vi "img test14(coutsegment attempt2).vi"() -> ()   [LabVIEW 2013]
uses:
  <vilib>/vision/NI_Vision_Development_Module.lvlib
panel:
  out "Top player court segment display 2":bool[][](array[boolean])
  out "count top":i32[](graph)
  out "count bottom":i32[](graph)
  out "trans top":i32[](graph)
  out "trans bottom":i32[](graph)
  out "trans array bottom":i32[](array[numeric])
  out "trans array top":i32[](array[numeric])
  out "count array bottom":i32[](array[numeric])
  out "Count array top":i32[](array[numeric])
  in  "ON":bool
  out "Top player court segment display":bool[][](array[boolean])
  out "bottom player":cluster{"Numeric":dbl, "Numeric":dbl}[](array[cluster])
  out "top player":cluster{"Numeric":dbl, "Numeric":dbl}[](array[cluster])
  in  "playing":bool
  out "Top VIew":cluster{"Numeric":dbl, "Numeric":dbl}[](graph)
  out "Image 4":T1(plugin-control)
  in  "frame jump":i32=3
  in  "speed":u32(slide)
  in  "start":i32(slide) step=219843704 scale=0.0..5867.0
  out "Image 3":T1(plugin-control)
  in  "AVI Path":path=path "E:/PhD work/Videos/ChenJin vs HuYun.avi"
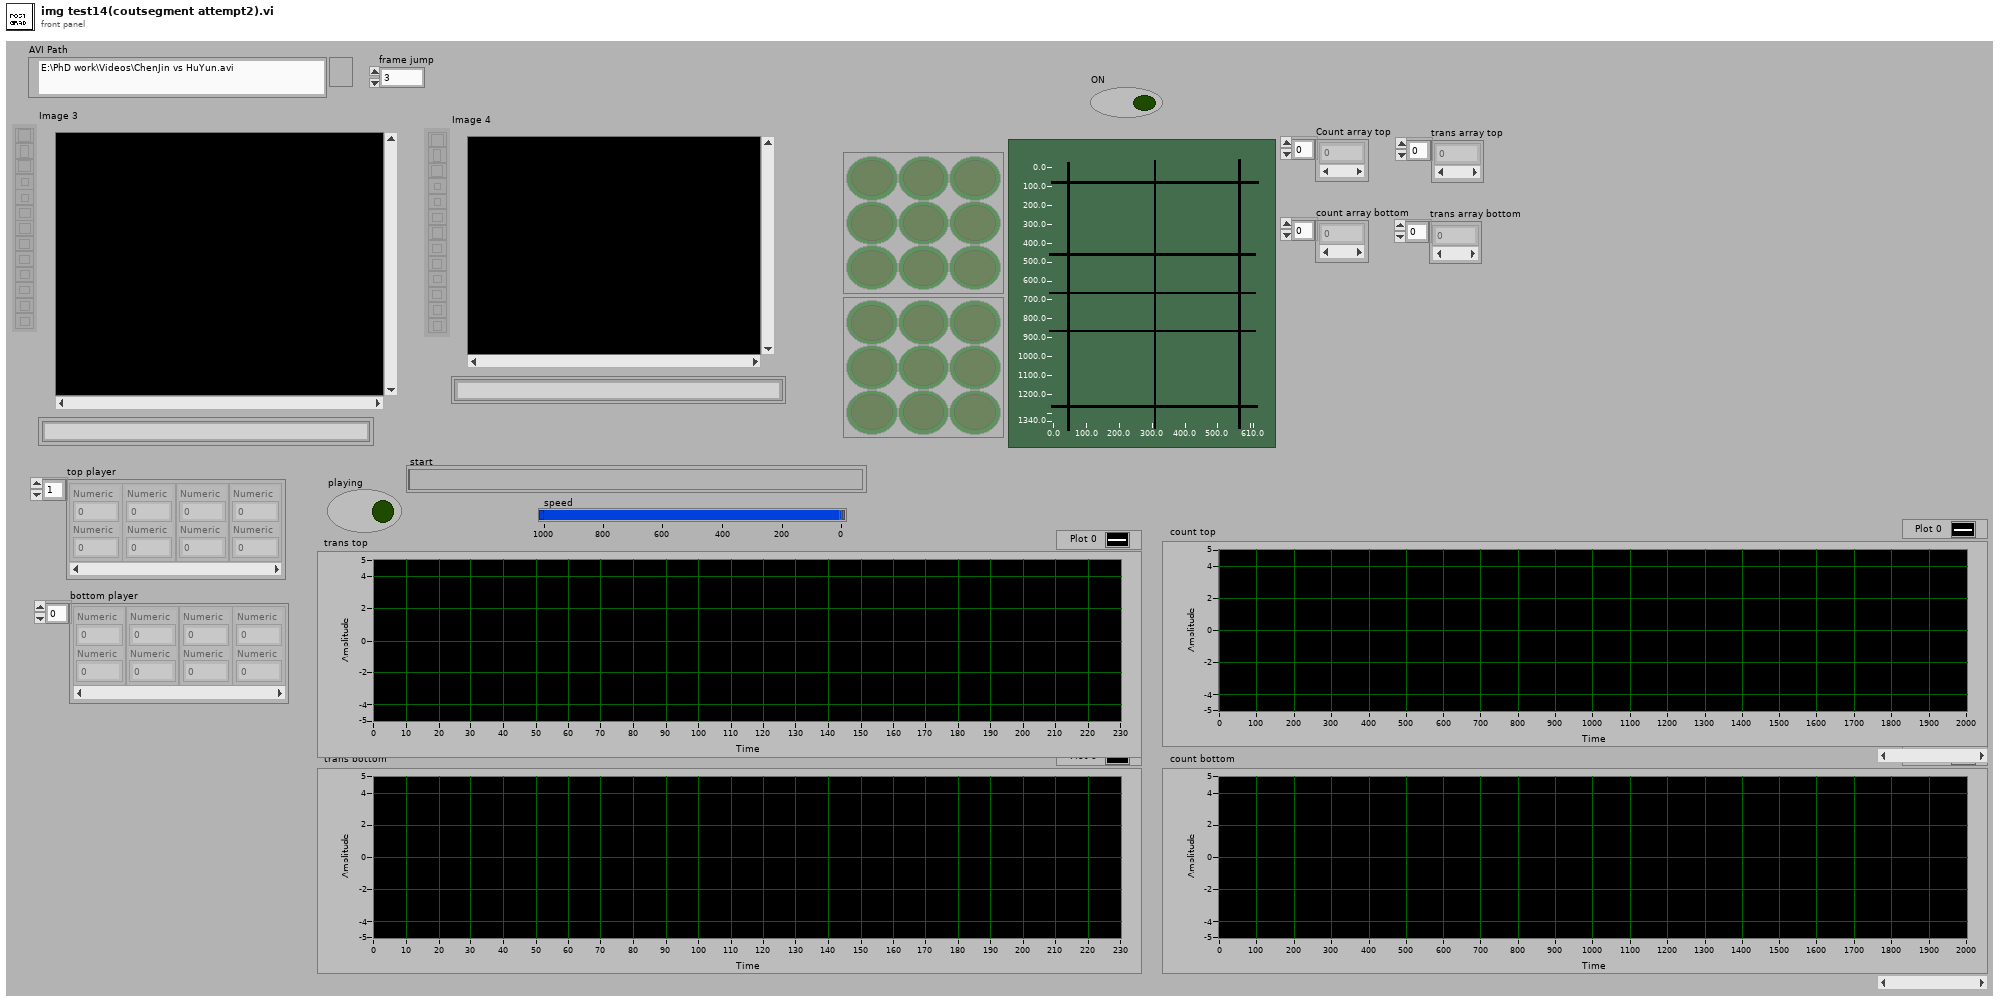
[diagram p1: front panel]
types:
  T1 = typedef "IMAQ Image.ctl" = refnum<image>
  T2 = cluster{cluster{"X":sgl, "Y":sgl}[], cluster{i32, i32}[], "Unit":u32}
  T3 = typedef "Image Type" = u32
  T4 = typedef "AviRefnum.ctl" = refnum<k1>
  T5 = cluster{"width":u32, "height":u32, "framesPerSecond":u32, "compressionFilter":string, "hasData":bool}
  T6 = cluster{"Origin Pixel":cluster{"X":sgl, "Y":sgl}, "Angle Relative to Horizontal (deg)":sgl, "Axis Reference":u32}
  T7 = typedef "Particle Parameters" = i32
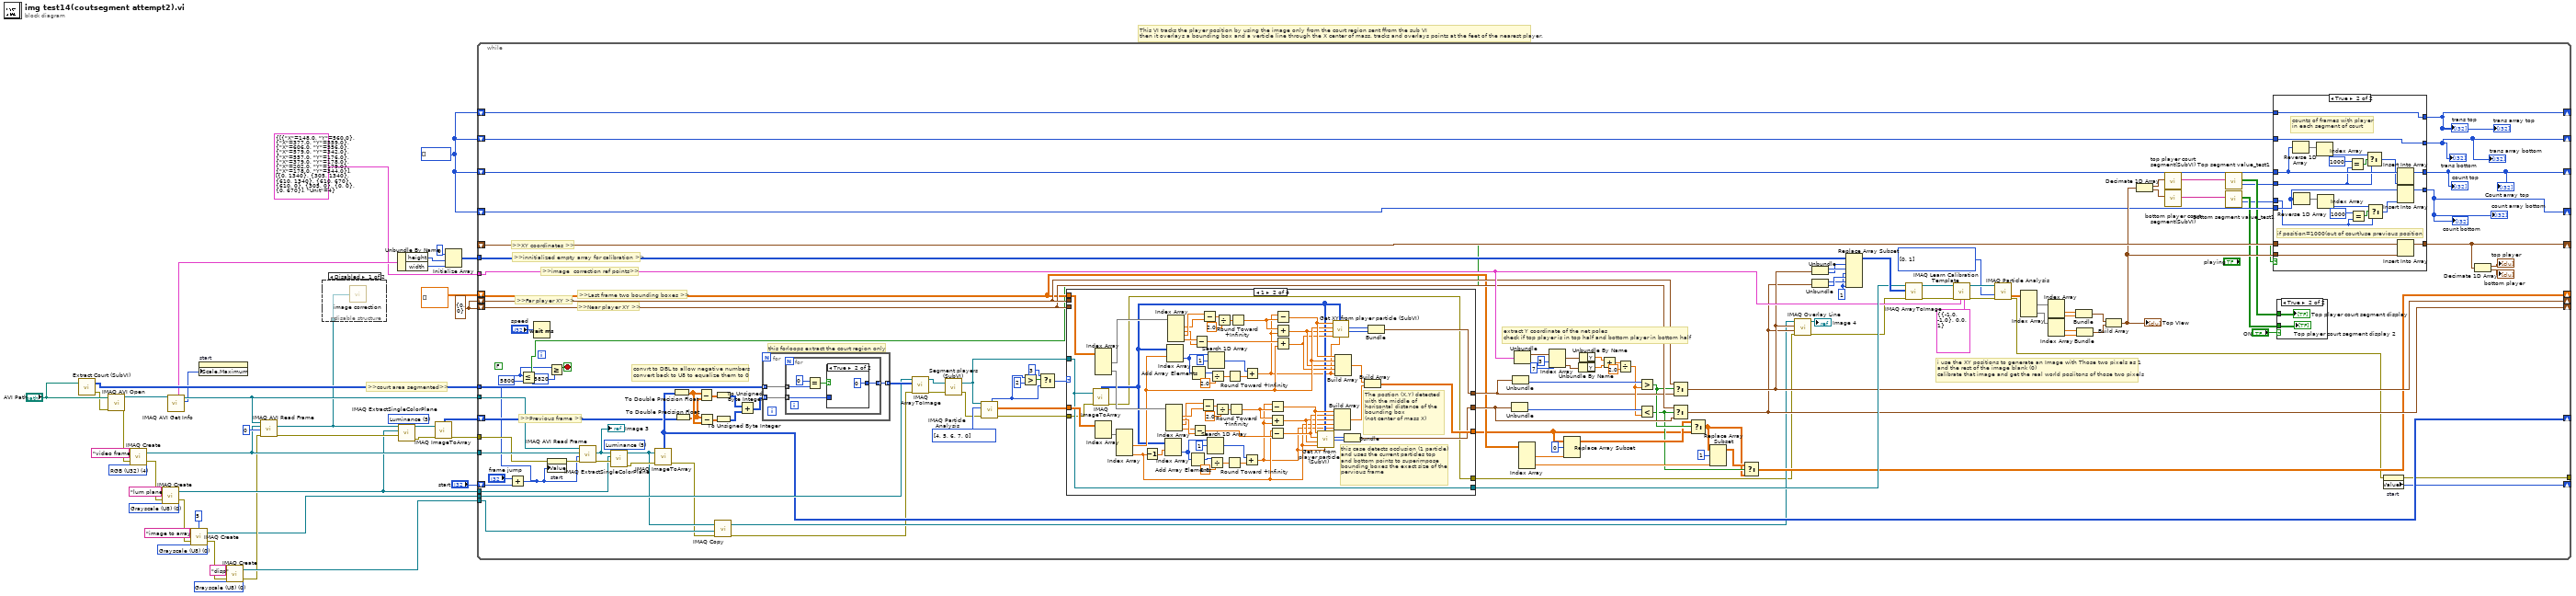
[diagram p0: block diagram]
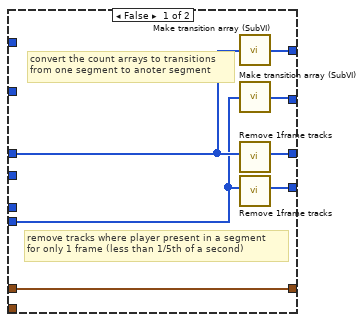
[diagram p3: hidden frame]
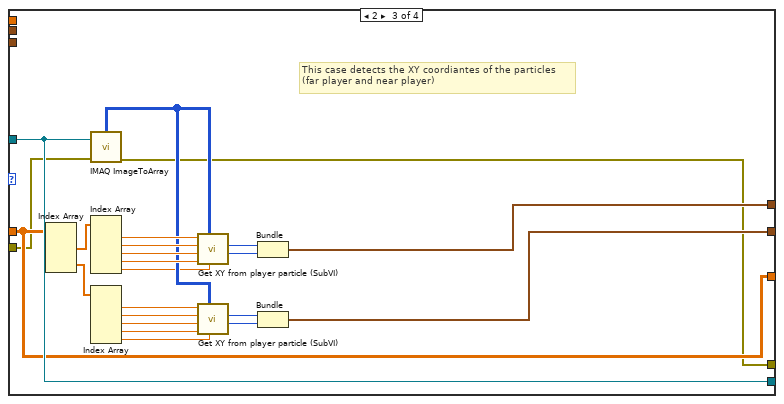
[diagram p6: hidden frame]
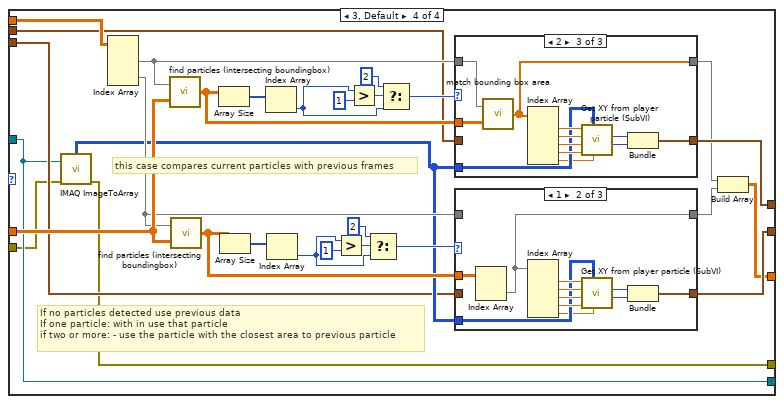
[diagram p7: hidden frame]
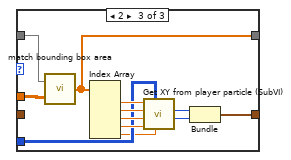
[diagram p9: hidden frame]
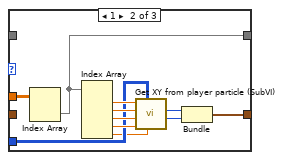
[diagram p11: hidden frame]
diagram:
  w2 = i32[] [] ("input array")
  w14 = cluster{"X coordinate":i32, "Y coordinate":i32} {"X coordinate"=0, "Y coordinate"=0}
  w27 = T3 0 items=["Grayscale (U8)", "Grayscale (I16)", "Grayscale (SGL)", "Complex (CSG)", "RGB (U32)", "HSL (U32)", "RGB (U64)", "Grayscale (U16)"] ("Image Type")
  w34 = 5 items=["Red", "Green", "Blue", "Hue", "Saturation", "Luminance", "Value", "Intensity"] ("Color Plane")
  w35 = T3 0 items=["Grayscale (U8)", "Grayscale (I16)", "Grayscale (SGL)", "Complex (CSG)", "RGB (U32)", "HSL (U32)", "RGB (U64)", "Grayscale (U16)"] ("Image Type")
  w39 = T3 0 items=["Grayscale (U8)", "Grayscale (I16)", "Grayscale (SGL)", "Complex (CSG)", "RGB (U32)", "HSL (U32)", "RGB (U64)", "Grayscale (U16)"] ("Image Type")
  w37 = T3 4 items=["Grayscale (U8)", "Grayscale (I16)", "Grayscale (SGL)", "Complex (CSG)", "RGB (U32)", "HSL (U32)", "RGB (U64)", "Grayscale (U16)"] ("Image Type")
  # ">>court area segmented>>"
  # "This VI tracks the player position by using the image only from the court region sent ffrom the sub VI\nthen it overlays a bounding box and a verticle line through the X center of mass. tracks and overlays points at the feet of the nearest player."
  n1 = call "Extract Court (SubVI).vi"("AVI Path"="AVI Path") -> ("error out"=w41:errorcluster, "Court pixels out"=w17:u8[][])  [unwired: 1 in]
  n2 = call "IMAQ AVI Open"("error in (no error)"=w41, "AVI Path"="AVI Path") -> ("error out"=w23:errorcluster, "Avi Refnum"=w12:T4)  [unwired: 8 in]
  n3 = call "IMAQ Create"("Image Name"="video frame", "Image Type"=w37, "error in (no error)"=w23) -> ("New Image"=w31:T1, "error out"=w22:errorcluster)  [unwired: 2 in]
  n4 = call "IMAQ Create"("Image Name"="lum plane", "Image Type"=w39, "error in (no error)"=w22) -> ("New Image"=w30:T1, "error out"=w21:errorcluster)  [unwired: 2 in]
  n5 = call "IMAQ AVI Get Info"("Avi Refnum"=w12) -> ("Number of Frames"=w10:u32, "Avi Refnum (duplicate)"=w11:T4, "Frame Data"=w7:T5)  [unwired: 6 in, 2 out]
  n6 = call "IMAQ Create"("Border Size"=5, "Image Name"="image to array", "Image Type"=w35, "error in (no error)"=w21) -> ("New Image"=w16:T1, "error out"=w20:errorcluster)  [unwired: 1 in]
  n7 = property on="start" class="Slide (strict)"("Scale.Maximum"=w10) -> ()  [unwired: 2 in, 2 out]
  n8 = call "IMAQ Create"("Image Name"="disp", "Image Type"=w27, "error in (no error)"=w20) -> ("New Image"=w25:T1, "error out"=w19:errorcluster)  [unwired: 2 in]
  n9 = call "IMAQ AVI Read Frame"("error in (no error)"=w19, "Frame Number"=u32 0, "Image"=w31, "Avi Refnum"=w11) -> ("error out"=w33:errorcluster, "Image Out"=w3:T1)  [unwired: 4 in, 2 out]
  n10 = disable-structure shown="Disabled" {
    disable-tunnel: w3 -> [w43 _]
    frame Disabled {
      n11 = call "image correction.vi"("Image"=w43) -> ()  [unwired: 1 out]
    }
    frame Enabled {
    }
  }
  n12 = Unbundle By Name(w7) -> ("height"=w6:u32, "width"=w5:u32)
  n13 = call "IMAQ ExtractSingleColorPlane"("Color Plane"=w34, "error in (no error)"=w33, "Image Dst"=w30, "Image Src"=w3) -> ("error out"=w24:errorcluster, "Image Dst Out"=w28:T1)  [unwired: 6 in]
  n14 = call "IMAQ ImageToArray"("error in (no error)"=w24, "Image"=w28) -> ("error out"=w9:errorcluster, "Image Pixels (U8)"=w29:u8[][])  [unwired: 2 in, 3 out]
  n15 = Initialize Array(u8 0 ("element"), w6, w5) -> (w4:u8[][])
  n16 = while {
    tunnel: w11 -> [w135]
    tunnel: w31 -> [w154]
    tunnel: w17 -> [w169]
    tunnel: w30 -> [w155]
    tunnel: w16 -> [w167]
    shift-right: [w166] -> _
    shift-left: w29 -> [w165]
    tunnel: w25 -> [w138]
    shift-right: [w76] -> _
    shift-left: dbl[][] [] ("Particle Measurements (Pixels)") -> [w86]
    shift-right: [w90] -> _
    shift-left: w14 -> [w92]
    shift-right: [w88] -> _
    shift-left: w14 -> [w91]
    shift-right: [w132] -> _
    shift-left: "start" -> [w137]
    tunnel: w9 -> [w134]
    tunnel: w4 -> [w131]
    tunnel: T2 {[{"X"=148.0, "Y"=560.0}, {"X"=377.0, "Y"=559.0}, {"X"=606.0, "Y"=556.0}, {"X"=579.0, "Y"=342.0}, {"X"=557.0, "Y"=176.0}, {"X"=379.0, "Y"=178.0}, {"X"=202.0, "Y"=179.0}, {"X"=178.0, "Y"=344.0}], [{0, 1340}, {305, 1340}, {610, 1340}, {610, 670}, {610, 0}, {305, 0}, {0, 0}, {0, 670}], "Unit"=4} ("ref points") -> [w105]
    shift-right: [w59] -> _
    shift-left: _ -> [w110]
    shift-right: [w56] -> _
    shift-left: w2 -> [w62]
    shift-right: [w55] -> _
    shift-left: w2 -> [w63]
    tunnel: [w65] -> _
    shift-right: [w57] -> _
    shift-left: w2 -> [w60]
    shift-right: [w58] -> _
    shift-left: w2 -> [w61]
    stop <- w46 stop-if-true
    w118 = T7[] [0, 1] items=["Center of Mass X", "Center of Mass Y", "First Pixel X", "First Pixel Y", "Bounding Rect Left", "Bounding Rect Top", "Bounding Rect Right", "Bounding Rect Bottom", "Max Feret Diameter Start X", "Max Feret Diameter Start Y", "Max Feret Diameter End X", "Max Feret Diameter End Y", "Max Horiz. Segment Length Left", "Max Horiz. Segment Length Right", "Max Horiz. Segment Length Row", "-", "Bounding Rect Width", "Bounding Rect Height", "Bounding Rect Diagonal", "Perimeter", "Convex Hull Perimeter", "Holes' Perimeter", "Max Feret Diameter", "Equivalent Ellipse Major Axis", "Equivalent Ellipse Minor Axis", "Equivalent Ellipse Minor Axis (Feret)", "Equivalent Rect Long Side", "Equivalent Rect Short Side", "Equivalent Rect Diagonal", "Equivalent Rect Short Side (Feret)", "Average Horiz. Segment Length", "Average Vert. Segment Length", "Hydraulic Radius", "Waddel Disk Diameter", "-", "Area", "Holes' Area", "Particle & Holes' Area", "Convex Hull Area", "Image Area", "-", "Number of Holes", "Number of Horiz. Segments", "Number of Vert. Segments", "-", "Orientation", "Max Feret Diameter Orientation", "-", "% Area/Image Area", "% Area/(Particle & Holes' Area)", "Ratio of Equivalent Ellipse Axes", "Ratio of Equivalent Rect Sides", "-", "Elongation Factor", "Compactness Factor", "Heywood Circularity Factor", "Type Factor", "-", "Sum X", "Sum Y", "Sum XX", "Sum XY", "Sum YY", "Sum XXX", "Sum XXY", "Sum XYY", "Sum YYY", "-", "Moment of Inertia XX", "Moment of Inertia XY", "Moment of Inertia YY", "Moment of Inertia XXX", "Moment of Inertia XXY", "Moment of Inertia XYY", "Moment of Inertia YYY", "Norm. Moment of Inertia XX", "Norm. Moment of Inertia XY", "Norm. Moment of Inertia YY", "Norm. Moment of Inertia XXX", "Norm. Moment of Inertia XXY", "Norm. Moment of Inertia XYY", "Norm. Moment of Inertia YYY", "Hu Moment 1", "Hu Moment 2", "Hu Moment 3", "Hu Moment 4", "Hu Moment 5", "Hu Moment 6", "Hu Moment 7"] ("Real-World Measurements")
    w126 = u8 1 ("new element/subarray")
    w156 = T7[] [4, 5, 6, 7, 0] items=["Center of Mass X", "Center of Mass Y", "First Pixel X", "First Pixel Y", "Bounding Rect Left", "Bounding Rect Top", "Bounding Rect Right", "Bounding Rect Bottom", "Max Feret Diameter Start X", "Max Feret Diameter Start Y", "Max Feret Diameter End X", "Max Feret Diameter End Y", "Max Horiz. Segment Length Left", "Max Horiz. Segment Length Right", "Max Horiz. Segment Length Row", "-", "Bounding Rect Width", "Bounding Rect Height", "Bounding Rect Diagonal", "Perimeter", "Convex Hull Perimeter", "Holes' Perimeter", "Max Feret Diameter", "Equivalent Ellipse Major Axis", "Equivalent Ellipse Minor Axis", "Equivalent Ellipse Minor Axis (Feret)", "Equivalent Rect Long Side", "Equivalent Rect Short Side", "Equivalent Rect Diagonal", "Equivalent Rect Short Side (Feret)", "Average Horiz. Segment Length", "Average Vert. Segment Length", "Hydraulic Radius", "Waddel Disk Diameter", "-", "Area", "Holes' Area", "Particle & Holes' Area", "Convex Hull Area", "Image Area", "-", "Number of Holes", "Number of Horiz. Segments", "Number of Vert. Segments", "-", "Orientation", "Max Feret Diameter Orientation", "-", "% Area/Image Area", "% Area/(Particle & Holes' Area)", "Ratio of Equivalent Ellipse Axes", "Ratio of Equivalent Rect Sides", "-", "Elongation Factor", "Compactness Factor", "Heywood Circularity Factor", "Type Factor", "-", "Sum X", "Sum Y", "Sum XX", "Sum XY", "Sum YY", "Sum XXX", "Sum XXY", "Sum XYY", "Sum YYY", "-", "Moment of Inertia XX", "Moment of Inertia XY", "Moment of Inertia YY", "Moment of Inertia XXX", "Moment of Inertia XXY", "Moment of Inertia XYY", "Moment of Inertia YYY", "Norm. Moment of Inertia XX", "Norm. Moment of Inertia XY", "Norm. Moment of Inertia YY", "Norm. Moment of Inertia XXX", "Norm. Moment of Inertia XXY", "Norm. Moment of Inertia XYY", "Norm. Moment of Inertia YYY", "Hu Moment 1", "Hu Moment 2", "Hu Moment 3", "Hu Moment 4", "Hu Moment 5", "Hu Moment 6", "Hu Moment 7"] ("Pixel Measurements")
    (unwired) FALSE
    w170 = 5 items=["Red", "Green", "Blue", "Hue", "Saturation", "Luminance", "Value", "Intensity"] ("Color Plane")
    # ">>XY coordinates >>"
    # ">>innitialized empty array for calibration >>"
    # ">>image  correction ref points>>"
    # "extract Y coordinate of the net poles\ncheck if top player is in top half and bottom player in bottom half"
    # "i use the XY positions to generate an Image with Those two pixels as 1 \nand the rest of the image blank (0)\ncalibrate that image and get the real world posiitons of those two pixels"
    # ">>Last frame two bounding boxes >>"
    # ">>Far player XY >>"
    # ">>Near player XY >>"
    # ">>Previous frame >>"
    # "convrt to DBL to allow negative numbers\nconvert back to U8 to equalize them to 0"
    # "this forloops extract the court region only"
    n17 = Add(x="frame jump", y=w137) -> (x+y=w45:i32)
    n18 = Less Or Equal?(x=w45, y=5800) -> (x <= y?=w47:bool)
    n19 = Wait (ms)(milliseconds to wait="speed") -> ()  [unwired: 1 out]
    n20 = property on="start" class="Slide (strict)"(error in=w134, "Value"=w45) -> (error out=w133:errorcluster)  [unwired: 1 in, 1 out]
    n21 = Greater Or Equal?(x=w45, y=5820) -> (x >= y?=w46:bool)
    n22 = call "IMAQ AVI Read Frame"("error in (no error)"=w133, "Frame Number"=w45, "Image"=w154, "Avi Refnum"=w135) -> ("error out"=w171:errorcluster, "Image Out"=w151:T1)  [unwired: 4 in, 2 out]
    "Image 3" <- w151
    n23 = call "IMAQ ExtractSingleColorPlane"("Color Plane"=w170, "error in (no error)"=w171, "Image Dst"=w155, "Image Src"=w151) -> ("error out"=w157:errorcluster, "Image Dst Out"=w139:T1)  [unwired: 6 in]
    n24 = call "IMAQ ImageToArray"("error in (no error)"=w157, "Image"=w139) -> ("error out"=w70:errorcluster, "Image Pixels (U8)"=w166:u8[][])  [unwired: 2 in, 3 out]
    n25 = To Double Precision Float(number=w166) -> (double precision float=w161:dbl[][])
    n26 = To Double Precision Float(number=w165) -> (double precision float=w160:dbl[][])
    n27 = Subtract(x=w161, y=w160) -> (x-y=w159:dbl[][])
    n28 = Subtract(x=w160, y=w161) -> (x-y=w158:dbl[][])
    n29 = call "IMAQ Copy"("error in (no error)"=w70, "Image Dst"=w138, "Image Src"=w139) -> ("error out"=w69:errorcluster, "Image Dst Out"=w71:T1)  [unwired: 3 in]
    n30 = To Unsigned Byte Integer(number=w159) -> (unsigned 8bit integer=w164:u8[][])
    n31 = To Unsigned Byte Integer(number=w158) -> (unsigned 8bit integer=w163:u8[][])
    n32 = Add(x=w164, y=w163) -> (x+y=w162:u8[][])
    n33 = for {
      tunnel: w169 -> [w372] mode=indexing
      tunnel: [w371] -> w168 mode=indexing
      tunnel: w162 -> [w370] mode=indexing
      n34 = for {
        tunnel: w372 -> [w377] mode=indexing
        tunnel: [w374] -> w371 mode=indexing
        tunnel: w370 -> [w373] mode=indexing
        n35 = Equal?(x=u8 0, y=w377) -> (x = y?=w375:bool)
        n36 = case shown="True" w375 {
          tunnel: [w378 u8 0 ("x")] -> w374
          tunnel: w373 -> [w378 _]
          frame False {
          }
          frame True {
          }
        }
      }
    }
    n37 = call "IMAQ ArrayToImage"("error in (no error)"=w69, "Image Pixels (U8)"=w168, "Image"=w167) -> ("error out"=w152:errorcluster, "Image Out"=w153:T1)  [unwired: 7 in]
    n38 = call "Segment players (SubVI).vi"("error In"=w152, "Image In"=w153) -> ("error out"=w145:errorcluster, "Image Out"=w143:T1)
    n39 = call "IMAQ Particle Analysis"("error in (no error)"=w145, "Pixel Measurements"=w156, "Image"=w143) -> ("error out"=w144:errorcluster, "Particle Measurements (Pixels)"=w142:dbl[][], "Number of Particles"=w147:i32)  [unwired: 3 in, 3 out]
    n40 = Greater?(x=w147, y=2) -> (0:w150:bool)
    n41 = Select(t=3 ("y"), s=w150, f=w147) -> (s? t:f=w146:i32)
    n42 = case shown="1" w146 {
      tunnel: [w205 w232 w286 w296] -> w124
      tunnel: w142 -> [_ w267 w272 w316]
      tunnel: w144 -> [w202 w208 w269 w292]
      tunnel: w143 -> [w205 w232 w286 w296]
      tunnel: [w203 w216 w274 w298] -> w87
      tunnel: [w204 w223 w273 w297] -> w89
      tunnel: [w206 w233 w272 w293] -> w75
      tunnel: w86 -> [w206 w257 _ w319]
      tunnel: w92 -> [w204 _ _ w304]
      tunnel: w91 -> [w203 _ _ w299]
      tunnel: [w202 w207 w268 w291] -> w67
      frame 0 {
        # "This case identifies frames where no particles are detected and keeps the same values from the\nprevious frame"
      }
      frame 1 {
        # "The postion (X,Y) detected with the middle of \nhorizontal distance of the bounding box\n(not center of mass X)"
        # "this case detects occlusion (1 particle)\nand uses the current particles top \nand bottom points to superimpose \nbounding boxes the exact size of the \npervious frame"
        n43 = call "IMAQ ImageToArray"("error in (no error)"=w208, "Image"=w232) -> ("error out"=w207:errorcluster, "Image Pixels (U8)"=w215:u8[][])  [unwired: 2 in, 3 out]
        n44 = Index Array(array=w257) -> (element #1=w265:dbl[], element #2=w237:dbl[])  [unwired: 4 in]
        n45 = Index Array(array=w267) -> (element=w266:dbl[])  [unwired: 2 in]
        n46 = Index Array(array=w266) -> (element #2=w228:dbl, element #4=w219:dbl)  [unwired: 4 in, 2 out]
        n47 = Decrement(x=w219) -> (x-1=w230:dbl)
        n48 = Index Array(array=w215, index (row)=w230) -> (element=w252:u8[])  [unwired: 1 in]
        n49 = Index Array(array=w237) -> (element #1=w241:dbl, element #2=w244:dbl, element #3=w240:dbl, element #4=w243:dbl)  [unwired: 4 in]
        n50 = Index Array(array=w215, index (row)=w228) -> (element=w245:u8[])  [unwired: 1 in]
        n51 = Index Array(array=w265) -> (element #1=w261:dbl, element #2=w258:dbl, element #3=w262:dbl, element #4=w259:dbl)  [unwired: 4 in]
        n52 = Add Array Elements(numeric array=w252) -> (sum=w253:u8)
        n53 = Add Array Elements(numeric array=w245) -> (sum=w249:u8)
        n54 = Subtract(x=w243, y=w244) -> (x-y=w231:dbl)
        n55 = Subtract(x=w259, y=w258) -> (x-y=w236:dbl)
        n56 = Subtract(x=w240, y=w241) -> (x-y=w239:dbl)
        n57 = Subtract(x=w262, y=w261) -> (x-y=w263:dbl)
        n58 = Search 1D Array(1D array=w252, element=u8 1) -> (index of element=w251:i32)  [unwired: 1 in]
        n59 = Search 1D Array(1D array=w245, element=u8 1) -> (index of element=w250:i32)  [unwired: 1 in]
        n60 = Divide(x=w253, y=2.0) -> (x/y=w254:dbl)
        n61 = Divide(x=w249, y=2.0) -> (x/y=w248:dbl)
        n62 = Divide(x=w239, y=2.0) -> (x/y=w242:dbl)
        n63 = Divide(x=w263, y=2.0) -> (x/y=w260:dbl)
        n64 = Round Toward +Infinity(x=w254) -> (ceil(x): smallest int >= x=w213:dbl)
        n65 = Round Toward +Infinity(x=w248) -> (ceil(x): smallest int >= x=w212:dbl)
        n66 = Round Toward +Infinity(x=w242) -> (ceil(x): smallest int >= x=w214:dbl)
        n67 = Round Toward +Infinity(x=w260) -> (ceil(x): smallest int >= x=w211:dbl)
        n68 = Add(x=w251, y=w213) -> (x+y=w209:dbl)
        n69 = Add(x=w250, y=w212) -> (x+y=w210:dbl)
        n70 = Subtract(x=w209, y=w214) -> (x-y=w222:dbl)
        n71 = Add(x=w214, y=w209) -> (x+y=w220:dbl)
        n72 = Subtract(x=w219, y=w231) -> (x-y=w221:dbl)
        n73 = Subtract(x=w210, y=w211) -> (x-y=w229:dbl)
        n74 = Add(x=w211, y=w210) -> (x+y=w227:dbl)
        n75 = Add(x=w236, y=w228) -> (x+y=w226:dbl)
        n76 = call "Get XY from player particle (SubVI).vi"("Center of mass X"=w209, "Image in Pixels (U8)"=w215, "Particle bounding rect bottom"=w219, "Particle bounding rect right"=w220, "Particle bounding rect top"=w221, "Particle bounding rect left"=w222) -> ("Y coordinate"=w217:i32, "X coordinate"=w218:i32)  [unwired: 2 in]
        n77 = call "Get XY from player particle (SubVI).vi"("Center of mass X"=w210, "Image in Pixels (U8)"=w215, "Particle bounding rect bottom"=w226, "Particle bounding rect right"=w227, "Particle bounding rect top"=w228, "Particle bounding rect left"=w229) -> ("Y coordinate"=w224:i32, "X coordinate"=w225:i32)  [unwired: 2 in]
        n78 = Build Array(w222, w221, w220, w219, w209) -> (w234:dbl[])
        n79 = Build Array(w229, w228, w227, w226, w210) -> (w235:dbl[])
        n80 = Bundle("X coordinate"=w218, "Y coordinate"=w217) -> (w216:cluster{"X coordinate":i32, "Y coordinate":i32})  [unwired: 1 in]
        n81 = Build Array(w235, w234) -> (w233:dbl[][])
        n82 = Bundle("X coordinate"=w225, "Y coordinate"=w224) -> (w223:cluster{"X coordinate":i32, "Y coordinate":i32})  [unwired: 1 in]
      }
      frame 2 {
        # "This case detects the XY coordiantes of the particles\n(far player and near player)"
        n83 = Index Array(array=w272) -> (element #1=w280:dbl[], element #2=w279:dbl[])  [unwired: 4 in]
        n84 = call "IMAQ ImageToArray"("error in (no error)"=w269, "Image"=w286) -> ("error out"=w268:errorcluster, "Image Pixels (U8)"=w281:u8[][])  [unwired: 2 in, 3 out]
        n85 = Index Array(array=w280) -> (element #1=w290:dbl, element #2=w289:dbl, element #3=w288:dbl, element #4=w287:dbl, element #5=w271:dbl)  [unwired: 5 in]
        n86 = Index Array(array=w279) -> (element #1=w282:dbl, element #2=w283:dbl, element #3=w284:dbl, element #4=w285:dbl, element #5=w270:dbl)  [unwired: 5 in]
        n87 = call "Get XY from player particle (SubVI).vi"("Center of mass X"=w271, "Image in Pixels (U8)"=w281, "Particle bounding rect bottom"=w287, "Particle bounding rect right"=w288, "Particle bounding rect top"=w289, "Particle bounding rect left"=w290) -> ("Y coordinate"=w277:i32, "X coordinate"=w278:i32)  [unwired: 2 in]
        n88 = call "Get XY from player particle (SubVI).vi"("Center of mass X"=w270, "Image in Pixels (U8)"=w281, "Particle bounding rect bottom"=w285, "Particle bounding rect right"=w284, "Particle bounding rect top"=w283, "Particle bounding rect left"=w282) -> ("Y coordinate"=w275:i32, "X coordinate"=w276:i32)  [unwired: 2 in]
        n89 = Bundle("X coordinate"=w278, "Y coordinate"=w277) -> (w273:cluster{"X coordinate":i32, "Y coordinate":i32})  [unwired: 1 in]
        n90 = Bundle("X coordinate"=w276, "Y coordinate"=w275) -> (w274:cluster{"X coordinate":i32, "Y coordinate":i32})  [unwired: 1 in]
      }
      frame 3, Default {
        # "If no particles detected use previous data\nIf one particle: with in use that particle\nif two or more: - use the particle with the closest area to previous particle"
        # "this case compares current particles with previous frames"
        n91 = call "IMAQ ImageToArray"("error in (no error)"=w292, "Image"=w296) -> ("error out"=w291:errorcluster, "Image Pixels (U8)"=w300:u8[][])  [unwired: 2 in, 3 out]
        n92 = Index Array(array=w319) -> (element #1=w315:dbl[], element #2=w303:dbl[])  [unwired: 4 in]
        n93 = call "find particles (intersecting boundingbox).vi"("Particle Measurements in (bounding boxes)"=w316, "bounding box in"=w315) -> ("Particles within bounding box"=w314:dbl[][])
        n94 = call "find particles (intersecting boundingbox).vi"("Particle Measurements in (bounding boxes)"=w316, "bounding box in"=w303) -> ("Particles within bounding box"=w301:dbl[][])
        n95 = Array Size(array=w314) -> (size(s)=w318:i32[])
        n96 = Array Size(array=w301) -> (size(s)=w317:i32[])
        n97 = Index Array(array=w318) -> (element=w306:i32)  [unwired: 1 in]
        n98 = Index Array(array=w317) -> (element=w307:i32)  [unwired: 1 in]
        n99 = Greater?(x=w307, y=1) -> (0:w310:bool)
        n100 = Greater?(x=w306, y=1) -> (0:w311:bool)
        n101 = Select(t=2 ("y"), s=w310, f=w307) -> (s? t:f=w302:i32)
        n102 = Select(t=2 ("y"), s=w311, f=w306) -> (s? t:f=w305:i32)
        n103 = case shown="2" w305 {
          tunnel: w315 -> [w346 _ w361]
          tunnel: w314 -> [_ w357 w360]
          tunnel: [w346 w348 w359] -> w295
          tunnel: w300 -> [_ w350 w363]
          tunnel: [w345 w349 w362] -> w297
          tunnel: w304 -> [w345 _ _]
          frame 0, Default {
          }
          frame 1 {
            n104 = Index Array(array=w357) -> (element=w348:dbl[])  [unwired: 2 in]
            n105 = Index Array(array=w348) -> (element #1=w354:dbl, element #2=w353:dbl, element #3=w352:dbl, element #4=w351:dbl, element #5=w347:dbl)  [unwired: 5 in]
            n106 = call "Get XY from player particle (SubVI).vi"("Center of mass X"=w347, "Image in Pixels (U8)"=w350, "Particle bounding rect bottom"=w351, "Particle bounding rect right"=w352, "Particle bounding rect top"=w353, "Particle bounding rect left"=w354) -> ("Y coordinate"=w355:i32, "X coordinate"=w356:i32)  [unwired: 2 in]
            n107 = Bundle("X coordinate"=w356, "Y coordinate"=w355) -> (w349:cluster{"X coordinate":i32, "Y coordinate":i32})  [unwired: 1 in]
          }
          frame 2 {
            n108 = call "match bounding box area.vi"("particle measurements (bounding box)"=w360, "bounding box in"=w361) -> ("matching bounding box"=w359:dbl[])
            n109 = Index Array(array=w359) -> (element #1=w367:dbl, element #2=w366:dbl, element #3=w365:dbl, element #4=w364:dbl, element #5=w358:dbl)  [unwired: 5 in]
            n110 = call "Get XY from player particle (SubVI).vi"("Center of mass X"=w358, "Image in Pixels (U8)"=w363, "Particle bounding rect bottom"=w364, "Particle bounding rect right"=w365, "Particle bounding rect top"=w366, "Particle bounding rect left"=w367) -> ("Y coordinate"=w368:i32, "X coordinate"=w369:i32)  [unwired: 2 in]
            n111 = Bundle("X coordinate"=w369, "Y coordinate"=w368) -> (w362:cluster{"X coordinate":i32, "Y coordinate":i32})  [unwired: 1 in]
          }
        }
        n112 = case shown="1" w302 {
          tunnel: w303 -> [w321 _ w336]
          tunnel: w301 -> [_ w332 w335]
          tunnel: [w321 w323 w334] -> w294
          tunnel: w300 -> [_ w325 w338]
          tunnel: [w320 w324 w337] -> w298
          tunnel: w299 -> [w320 _ _]
          frame 0, Default {
          }
          frame 1 {
            n113 = Index Array(array=w332) -> (element=w323:dbl[])  [unwired: 2 in]
            n114 = Index Array(array=w323) -> (element #1=w329:dbl, element #2=w328:dbl, element #3=w327:dbl, element #4=w326:dbl, element #5=w322:dbl)  [unwired: 5 in]
            n115 = call "Get XY from player particle (SubVI).vi"("Center of mass X"=w322, "Image in Pixels (U8)"=w325, "Particle bounding rect bottom"=w326, "Particle bounding rect right"=w327, "Particle bounding rect top"=w328, "Particle bounding rect left"=w329) -> ("Y coordinate"=w330:i32, "X coordinate"=w331:i32)  [unwired: 2 in]
            n116 = Bundle("X coordinate"=w331, "Y coordinate"=w330) -> (w324:cluster{"X coordinate":i32, "Y coordinate":i32})  [unwired: 1 in]
          }
          frame 2 {
            n117 = call "match bounding box area.vi"("particle measurements (bounding box)"=w335, "bounding box in"=w336) -> ("matching bounding box"=w334:dbl[])
            n118 = Index Array(array=w334) -> (element #1=w342:dbl, element #2=w341:dbl, element #3=w340:dbl, element #4=w339:dbl, element #5=w333:dbl)  [unwired: 5 in]
            n119 = call "Get XY from player particle (SubVI).vi"("Center of mass X"=w333, "Image in Pixels (U8)"=w338, "Particle bounding rect bottom"=w339, "Particle bounding rect right"=w340, "Particle bounding rect top"=w341, "Particle bounding rect left"=w342) -> ("Y coordinate"=w343:i32, "X coordinate"=w344:i32)  [unwired: 2 in]
            n120 = Bundle("X coordinate"=w344, "Y coordinate"=w343) -> (w337:cluster{"X coordinate":i32, "Y coordinate":i32})  [unwired: 1 in]
          }
        }
        n121 = Build Array(w295, w294) -> (w293:dbl[][])
      }
    }
    n122 = Unbundle(w87) -> ("Y coordinate"=w94:i32)  [unwired: 1 out]
    n123 = Unbundle(w89) -> ("Y coordinate"=w95:i32)  [unwired: 1 out]
    n124 = Unbundle(w105) -> (w104:cluster{"X":sgl, "Y":sgl}[])  [unwired: 2 out]
    n125 = Index Array(array=w86) -> (element #1=w84:dbl[], element #2=w80:dbl[])  [unwired: 4 in]
    n126 = Index Array(array=w104, index #1=3 ("index"), index #2=7 ("index")) -> (element #1=w101:cluster{"X":sgl, "Y":sgl}, element #2=w100:cluster{"X":sgl, "Y":sgl})
    n127 = Replace Array Subset(array=w75, new element=w84, index (row)=0) -> (w83:dbl[][])  [unwired: 1 in]
    n128 = Unbundle By Name(w100) -> ("Y"=w98:sgl)
    n129 = Unbundle By Name(w101) -> ("Y"=w99:sgl)
    n130 = Add(x=w99, y=w98) -> (x+y=w97:sgl)
    n131 = Divide(x=w97, y=sgl 2.0) -> (x/y=w93:sgl)
    n132 = Greater?(x=w95, y=w93) -> (0:w85:bool)
    n133 = Less?(x=w94, y=w93) -> (x < y?=w78:bool)
    n134 = Select(t=w92, s=w85, f=w89) -> (s? t:f=w90:cluster{"X coordinate":i32, "Y coordinate":i32})
    n135 = Select(t=w91, s=w78, f=w87) -> (s? t:f=w88:cluster{"X coordinate":i32, "Y coordinate":i32})
    n136 = Select(t=w83, s=w85, f=w75) -> (s? t:f=w77:dbl[][])
    n137 = Replace Array Subset(array=w77, new element=w80, index (row)=1) -> (w79:dbl[][])  [unwired: 1 in]
    n138 = Select(t=w79, s=w78, f=w77) -> (s? t:f=w76:dbl[][])
    n139 = call "IMAQ Overlay Line"("error in (no error)"=w67, "End Point"=w88, "Start Point"=w90, "Image"=w71) -> ("error out"=w68:errorcluster, "Image Out"=→"Image 4":T1)  [unwired: 6 in]
    n140 = Unbundle(w88) -> ("X coordinate"=w127:i32, "Y coordinate"=w128:i32)
    n141 = Unbundle(w90) -> ("X coordinate"=w130:i32, "Y coordinate"=w129:i32)
    n142 = Replace Array Subset(array=w131, new element #1=w126, index (row) #1=w129, index (col) #1=w130, new element #2=w126, index (row) #2=w128, index (col) #2=w127) -> (w125:u8[][])
    n143 = call "IMAQ ArrayToImage"("error in (no error)"=w68, "Image Pixels (U8)"=w125, "Image"=w124) -> ("error out"=w121:errorcluster, "Image Out"=w122:T1)  [unwired: 7 in]
    n144 = call "IMAQ Learn Calibration Template"("Calibration Axis Info"=T6 {"Origin Pixel"={"X"=-1.0, "Y"=-1.0}, "Angle Relative to Horizontal (deg)"=0.0, "Axis Reference"=1}, "Reference Points"=w105, "error in (no error)"=w121, "Image"=w122) -> ("error out"=w120:errorcluster, "Calibrated Image"=w119:T1)  [unwired: 5 in, 1 out]
    n145 = call "IMAQ Particle Analysis"("error in (no error)"=w120, "Real-World Measurements"=w118, "Image"=w119) -> ("error out"=w66:errorcluster, "Particle Measurements (Real-World)"=w117:dbl[][])  [unwired: 3 in, 4 out]
    n146 = Index Array(array=w117) -> (element #1=w116:dbl[], element #2=w115:dbl[])  [unwired: 4 in]
    n147 = Index Array(array=w116) -> (element #1=w112:dbl, element #2=w111:dbl)  [unwired: 2 in]
    n148 = Index Array(array=w115) -> (element #1=w113:dbl, element #2=w114:dbl)  [unwired: 2 in]
    n149 = Bundle("Numeric"=w112, "Numeric"=w111) -> (w109:cluster{"Numeric":dbl, "Numeric":dbl})  [unwired: 1 in]
    n150 = Bundle("Numeric"=w113, "Numeric"=w114) -> (w108:cluster{"Numeric":dbl, "Numeric":dbl})  [unwired: 1 in]
    n151 = Build Array(w109, w108) -> (w74:cluster{"Numeric":dbl, "Numeric":dbl}[])
    "Top VIew" <- w74
    n152 = Decimate 1D Array(w74) -> (w72:cluster{"Numeric":dbl, "Numeric":dbl}[], w73:cluster{"Numeric":dbl, "Numeric":dbl}[])
    n153 = call "top player court segment(SubVI).vi"("Top player position"=w72) -> ("Top player segment position"=w50:string)  [unwired: 10 in]
    n154 = call "bottom player court segment(SubVI).vi"("Bottom player position"=w73) -> ("Bottom player segment position"=w49:string)  [unwired: 10 in]
    n155 = call "Top segment value_test1.vi"("Top player segment position"=w50) -> ("Top player segment value"=w53:i32, "Top player court segment display"=w54:bool[][])  [unwired: 9 in]
    n156 = call "Bottom segment value_test1.vi"("Bottom player segment position"=w49) -> ("Bottom player segment"=w51:i32, "Bottom player court segment display"=w52:bool[][])  [unwired: 9 in]
    n157 = case shown="True" w47 {
      tunnel: w110 -> [w178 w199]
      tunnel: w74 -> [_ w198]
      tunnel: w63 -> [w175 w192]
      tunnel: w62 -> [w172 w182]
      tunnel: [w173 w193] -> w57
      tunnel: [w174 w194] -> w58
      tunnel: w51 -> [_ w179]
      tunnel: w53 -> [_ w187]
      tunnel: w61 -> [_ w194]
      tunnel: w60 -> [_ w193]
      tunnel: [w176 w197] -> w56
      tunnel: [w177 w196] -> w55
      tunnel: [w178 w195] -> w59
      frame False {
        # "convert the count arrays to transitions \nfrom one segment to anoter segment"
        # "remove tracks where player present in a segment \nfor only 1 frame (less than 1/5th of a second)"
        n158 = call "Make transition array (SubVI).vi"("count array in"=w175) -> ("Transition array out"=w173:i32[])
        n159 = call "Make transition array (SubVI).vi"("count array in"=w172) -> ("Transition array out"=w174:i32[])
        n160 = call "Remove 1frame tracks.vi"("count array in"=w175) -> ("count array out"=w177:i32[])  [unwired: 10 in]
        n161 = call "Remove 1frame tracks.vi"("count array in"=w172) -> ("count array out"=w176:i32[])  [unwired: 10 in]
      }
      frame True {
        # "if position=1000(out of court)use previous position"
        # "counts of frames with player\nin each segment of court"
        n162 = Reverse 1D Array(array=w192) -> (reversed array=w191:i32[])
        n163 = Reverse 1D Array(array=w182) -> (reversed array=w181:i32[])
        n164 = Index Array(array=w191) -> (element=w188:i32)  [unwired: 1 in]
        n165 = Index Array(array=w181) -> (element=w185:i32)  [unwired: 1 in]
        n166 = Equal?(x=1000 ("y"), y=w187) -> (x = y?=w189:bool)
        n167 = Equal?(x=1000 ("y"), y=w179) -> (x = y?=w184:bool)
        n168 = Select(t=w188, s=w189, f=w187) -> (s? t:f=w186:i32)
        n169 = Select(t=w185, s=w184, f=w179) -> (s? t:f=w180:i32)
        n170 = Insert Into Array(array=w192, new element=w186) -> (w196:i32[])  [unwired: 1 in]
        n171 = Insert Into Array(array=w182, new element=w180) -> (w197:i32[])  [unwired: 1 in]
        n172 = Insert Into Array(array=w199, new element=w198) -> (w195:cluster{"Numeric":dbl, "Numeric":dbl}[])  [unwired: 1 in]
      }
    }
    "Count array top" <- w55
    "count array bottom" <- w56
    "trans array top" <- w57
    "trans array bottom" <- w58
    "trans bottom" <- w58
    "trans top" <- w57
    "count bottom" <- w56
    "count top" <- w55
    n173 = case shown="True" "ON" {
      tunnel: w54 -> [_ w201]
      tunnel: w52 -> [_ w200]
      frame False {
      }
      frame True {
        "Top player court segment display" <- w201
        "Top player court segment display 2" <- w200
      }
    }
    n174 = property on="start" class="Slide (strict)"(error in=w66) -> (error out=w65:errorcluster, "Value"=w132:i32)  [unwired: 1 in, 1 out]
    n175 = Decimate 1D Array(w59) -> (→"top player":cluster{"Numeric":dbl, "Numeric":dbl}[], →"bottom player":cluster{"Numeric":dbl, "Numeric":dbl}[])
  }
